vi "ViperHawk_Decode MC Data.vi"(10 "Array":u8[](array[numeric]), 11 "Diagnostic Data In":T1) -> (3 "Diagnostic Data Out":T1)   [LabVIEW 2016]
uses:
  Type Definitions/ViperHawk/ViperHawk Diagnostic Data.ctl
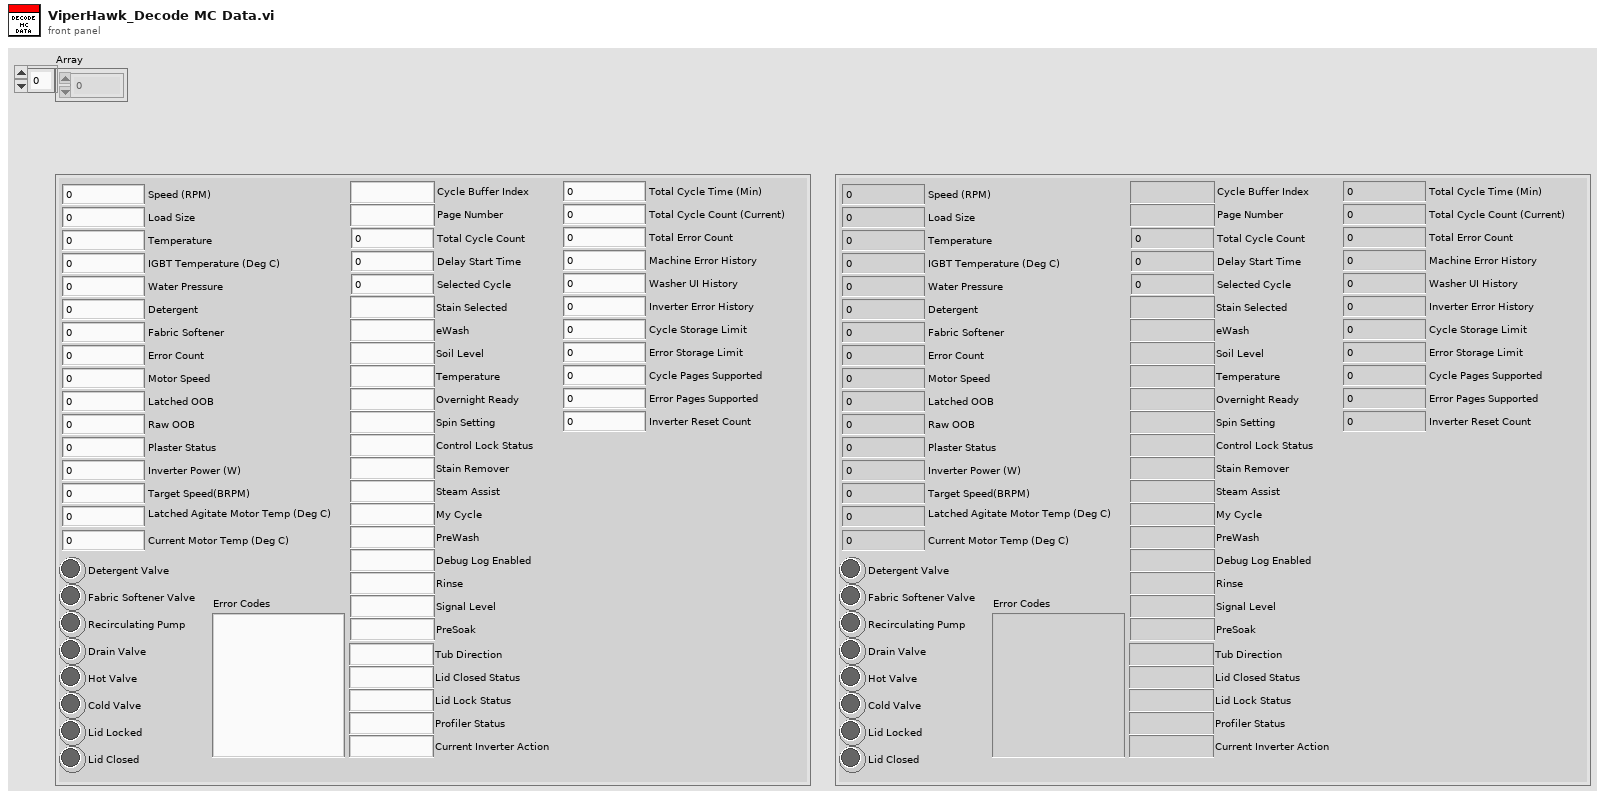
[diagram p1: front panel]
types:
  T1 = typedef "ViperHawk Diagnostic Data.ctl" = cluster{"Speed (RPM)":u32, "Load Size":u32, "Temperature":u32, "Water Pressure":dbl, "Detergent":u32, "Fabric Softener":u32, "Tub Direction":string, "Detergent Valve":bool, "Fabric Softener Valve":bool, "Recirculating Pump":bool, "Drain Valve":bool, "Hot Valve":bool, "Cold Valve":bool, "Lid Closed Status":string, "Lid Lock Status":string, "Error Count":u32, "IGBT Temperature (Deg C)":u32, "Motor Speed":u32, "Latched OOB":u32, "Raw OOB":u32, "Plaster Status":u32, "Inverter Power (W)":u32, "Target Speed(BRPM)":u32, "Latched Agitate Motor Temp (Deg C)":u32, "Current Motor Temp (Deg C)":u32, "Profiler Status":string, "Current Inverter Action":string, "Error Codes":string, "Lid Locked":bool, "Lid Closed":bool, "9E Diagnostic Data":cluster{"Total Cycle Time (Min)":u32, "Total Cycle Count (Current)":u16, "Total Error Count":u16, "Machine Error History":u32, "Washer UI History":u32, "Inverter Error History":u32, "Cycle Storage Limit":u8, "Error Storage Limit":u8, "Cycle Pages Supported":u8, "Error Pages Supported":u8, "Inverter Reset Count":u16}, "9F Diagnostic Data":cluster{"Cycle Buffer Index":string, "Page Number":string, "Total Cycle Count":u32, "Delay Start Time":u32, "Stain Selected":string, "Selected Cycle":u32, "eWash":string, "Soil Level":string, "Temperature":string, "Overnight Ready":string, "Spin Setting":string, "Control Lock Status":string, "Stain Remover":string, "Steam Assist":string, "My Cycle":string, "PreWash":string, "Debug Log Enabled":string, "Rinse":string, "Signal Level":string, "PreSoak":string}}
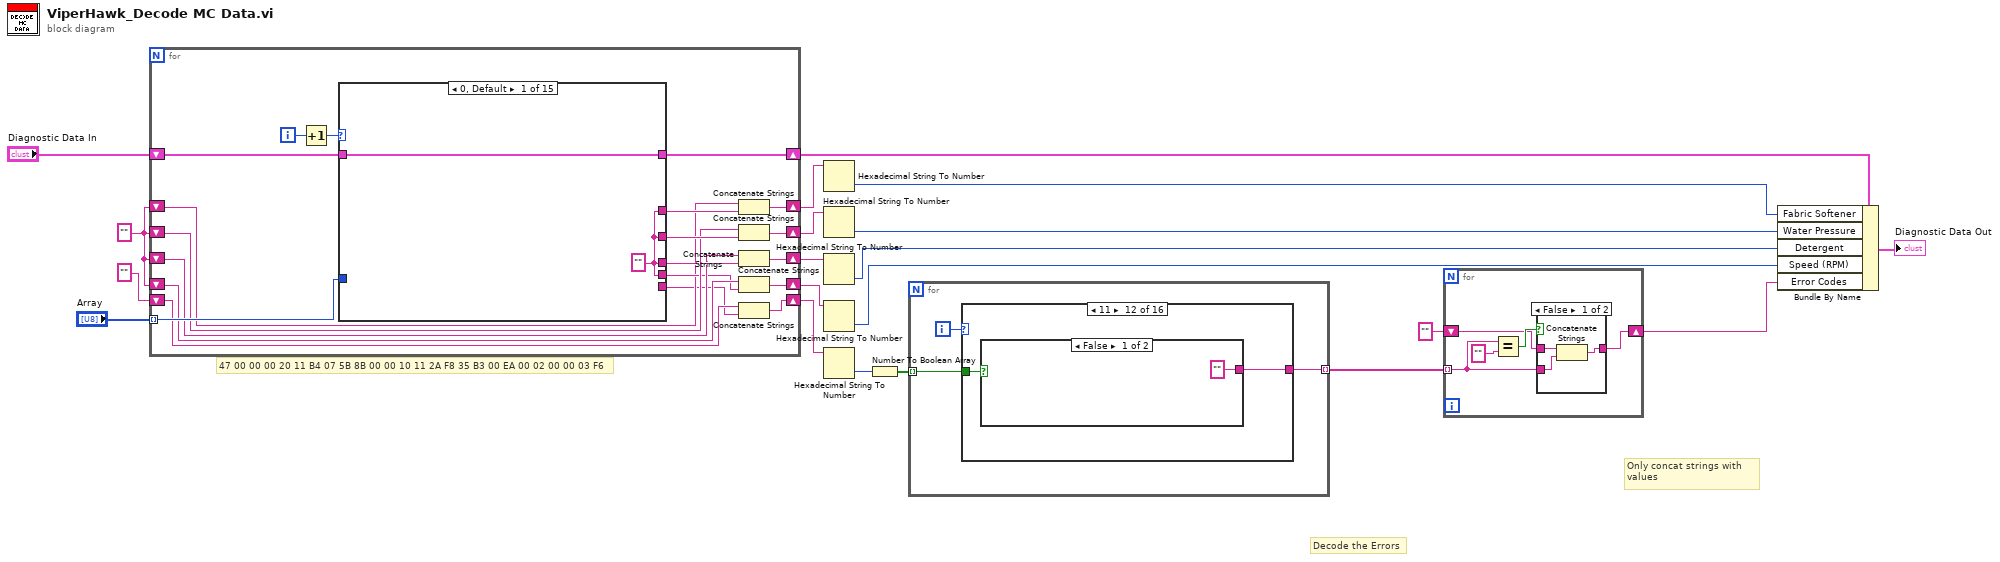
[diagram p0: block diagram]
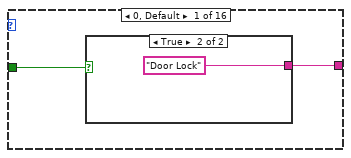
[diagram p3: hidden frame]
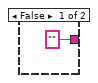
[diagram p4: hidden frame]
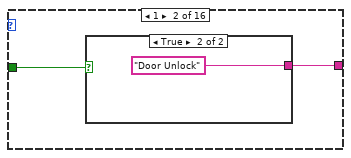
[diagram p5: hidden frame]
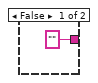
[diagram p6: hidden frame]
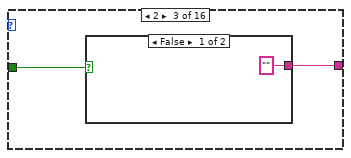
[diagram p7: hidden frame]
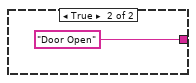
[diagram p8: hidden frame]
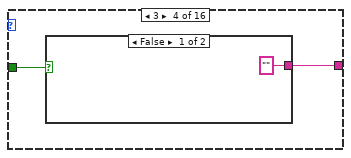
[diagram p9: hidden frame]
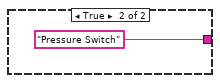
[diagram p10: hidden frame]
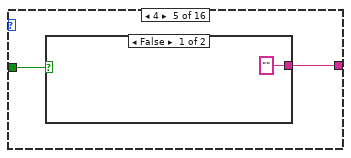
[diagram p11: hidden frame]
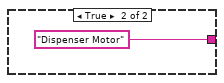
[diagram p12: hidden frame]
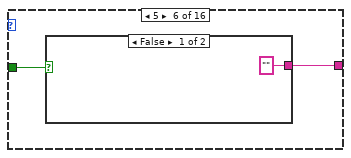
[diagram p13: hidden frame]
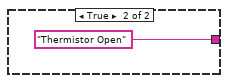
[diagram p14: hidden frame]
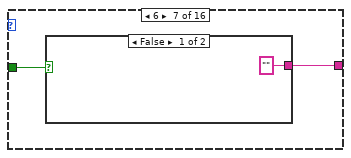
[diagram p15: hidden frame]
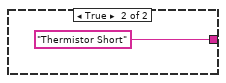
[diagram p16: hidden frame]
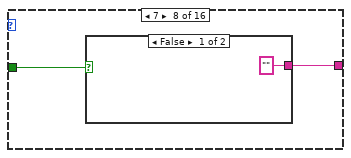
[diagram p17: hidden frame]
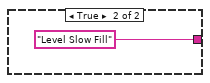
[diagram p18: hidden frame]
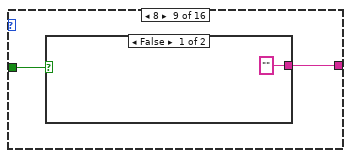
[diagram p19: hidden frame]
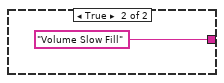
[diagram p20: hidden frame]
diagram:
  w16 = ""
  # "Only concat strings with \nvalues"
  # "Decode the Errors"
  # "47 00 00 00 20 11 B4 07 5B 8B 00 00 10 11 2A F8 35 B3 00 EA 00 02 00 00 03 F6"
  n1 = for {
    tunnel: "Array" -> [w40] mode=indexing
    shift-right: [w35] -> w19
    shift-left: w16 -> [w36]
    shift-right: [w34] -> w18
    shift-left: w16 -> [w32]
    shift-right: [w30] -> w20
    shift-left: w16 -> [w24]
    shift-right: [w29] -> w17
    shift-left: w16 -> [w28]
    shift-right: [w25] -> w15
    shift-left: "Diagnostic Data In" -> [w26]
    shift-right: [w21] -> w8
    shift-left: "" -> [w23]
    i -> [w38]
    n2 = Increment(x=w38) -> (x+1=w39:i32)
    n3 = case shown="0, Default" w39 {
      tunnel: w40 -> [_ w43 w51 w59 w63 w67 w73 w77 w80 w85 w89 w92 w96 w101 w105]
      tunnel: [w42 _ _ _ w62 w66 _ _ _ _ _ _ _ _ _] -> w37
      tunnel: [w42 _ _ _ _ _ _ w76 w79 _ _ _ _ _ _] -> w33
      tunnel: [w42 _ _ _ _ _ _ _ _ w84 w88 _ _ _ _] -> w31
      tunnel: [w42 _ _ _ _ _ _ _ _ _ _ _ _ w100 w104] -> w27
      tunnel: w26 -> [w41 w45 w49 w57 w61 w65 w71 w75 w81 w83 w87 w93 w97 w99 w103]
      tunnel: [w41 w44 w48 w56 w61 w65 w68 w75 w81 w83 w87 w93 w97 w99 w103] -> w25
      tunnel: [_ _ _ _ _ _ _ _ _ _ _ w91 w95 _ _] -> w22
      frame 0, Default {
        w42 = ""
      }
      frame 1 {
        n4 = Bundle By Name(cluster=w45, "Temperature"=w43) -> (w44:T1)
      }
      frame 4 {
        n5 = Number To Boolean Array(number=w51) -> (Boolean array=w50:bool[])
        n6 = Index Array(array=w50) -> (element #1=w47:bool, element #2=w46:bool)  [unwired: 2 in]
        n7 = Bundle By Name(cluster=w49, "Hot Valve"=w47, "Cold Valve"=w46) -> (w48:T1)
      }
      frame 5 {
        n8 = Number To Boolean Array(number=w59) -> (Boolean array=w58:bool[])
        n9 = Index Array(array=w58) -> (element #3=w55:bool, element #4=w54:bool, element #5=w53:bool, element #6=w52:bool)  [unwired: 6 in, 2 out]
        n10 = Bundle By Name(cluster=w57, "Detergent Valve"=w55, "Fabric Softener Valve"=w54, "Recirculating Pump"=w53, "Drain Valve"=w52) -> (w56:T1)
      }
      frame 6 {
        # "water pressure"
        n11 = Number To Hexadecimal String(1:i16 2 ("width (-)"), 2:w63) -> (0:w62:string)
      }
      frame 7 {
        # "water pressure"
        n12 = Number To Hexadecimal String(1:i16 2 ("width (-)"), 2:w67) -> (0:w66:string)
      }
      frame 10 {
        n13 = Number To Boolean Array(number=w73) -> (Boolean array=w72:bool[])
        n14 = Index Array(array=w72) -> (element #1=w70:bool, element #2=w69:bool)  [unwired: 2 in]
        n15 = Bundle By Name(cluster=w71, "Lid Closed"=w70, "Lid Locked"=w69) -> (w68:T1)
      }
      frame 15 {
        # "detergent"
        n16 = Number To Hexadecimal String(1:i16 2 ("width (-)"), 2:w77) -> (0:w76:string)
      }
      frame 16 {
        # "detergent"
        n17 = Number To Hexadecimal String(1:i16 2 ("width (-)"), 2:w80) -> (0:w79:string)
      }
      frame 17 {
        # "fs"
        n18 = Number To Hexadecimal String(1:i16 2 ("width (-)"), 2:w85) -> (0:w84:string)
      }
      frame 18 {
        # "fs"
        n19 = Number To Hexadecimal String(1:i16 2 ("width (-)"), 2:w89) -> (0:w88:string)
      }
      frame 21 {
        # "Error Code"
        n20 = Number To Hexadecimal String(1:i16 2 ("width (-)"), 2:w92) -> (0:w91:string)
      }
      frame 22 {
        # "Error Code"
        n21 = Number To Hexadecimal String(1:i16 2 ("width (-)"), 2:w96) -> (0:w95:string)
      }
      frame 25 {
        # "hall sensor"
        n22 = Number To Hexadecimal String(1:i16 2 ("width (-)"), 2:w101) -> (0:w100:string)
      }
      frame 26 {
        # "hall sensor"
        n23 = Number To Hexadecimal String(1:i16 2 ("width (-)"), 2:w105) -> (0:w104:string)
      }
    }
    n24 = Concatenate Strings(w24, w31) -> (w30:string)
    n25 = Concatenate Strings(w36, w37) -> (w35:string)
    n26 = Concatenate Strings(w32, w33) -> (w34:string)
    n27 = Concatenate Strings(w28, w27) -> (w29:string)
    n28 = Concatenate Strings(w23, w22) -> (w21:string)
  }
  n29 = Hexadecimal String To Number(string=w20) -> (number=w12:u32)  [unwired: 2 in, 1 out]
  n30 = Hexadecimal String To Number(string=w19) -> (number=w13:u32)  [unwired: 2 in, 1 out]
  n31 = Hexadecimal String To Number(string=w18) -> (number=w14:u32)  [unwired: 2 in, 1 out]
  n32 = Hexadecimal String To Number(string=w17) -> (number=w11:u32)  [unwired: 2 in, 1 out]
  n33 = Hexadecimal String To Number(string=w8) -> (number=w7:u32)  [unwired: 2 in, 1 out]
  n34 = Number To Boolean Array(number=w7) -> (Boolean array=w10:bool[])
  n35 = for {
    tunnel: w10 -> [w107] mode=indexing
    tunnel: [w106] -> w6 mode=indexing
    i -> [w108]
    n36 = case shown="11" w108 {
      tunnel: w107 -> [w110 w114 w118 w122 w126 w130 w134 w138 w141 w145 w149 w153 w157 w161 _ _]
      tunnel: [w109 w113 w117 w121 w125 w129 w133 w137 w142 w146 w150 w154 w158 w162 "" ""] -> w106
      frame 0, Default {
        n37 = case shown="True" w110 {
          tunnel: ["" "Door Lock"] -> w109
          frame False {
          }
          frame True {
          }
        }
      }
      frame 1 {
        n38 = case shown="True" w114 {
          tunnel: ["" "Door Unlock"] -> w113
          frame False {
          }
          frame True {
          }
        }
      }
      frame 2 {
        n39 = case shown="False" w118 {
          tunnel: ["" "Door Open"] -> w117
          frame False {
          }
          frame True {
          }
        }
      }
      frame 3 {
        n40 = case shown="False" w122 {
          tunnel: ["" "Pressure Switch"] -> w121
          frame False {
          }
          frame True {
          }
        }
      }
      frame 4 {
        n41 = case shown="False" w126 {
          tunnel: ["" "Dispenser Motor"] -> w125
          frame False {
          }
          frame True {
          }
        }
      }
      frame 5 {
        n42 = case shown="False" w130 {
          tunnel: ["" "Thermistor Open"] -> w129
          frame False {
          }
          frame True {
          }
        }
      }
      frame 6 {
        n43 = case shown="False" w134 {
          tunnel: ["" "Thermistor Short"] -> w133
          frame False {
          }
          frame True {
          }
        }
      }
      frame 7 {
        n44 = case shown="False" w138 {
          tunnel: ["" "Level Slow Fill"] -> w137
          frame False {
          }
          frame True {
          }
        }
      }
      frame 8 {
        n45 = case shown="False" w141 {
          tunnel: ["" "Volume Slow Fill"] -> w142
          frame False {
          }
          frame True {
          }
        }
      }
      frame 9 {
        n46 = case shown="False" w145 {
          tunnel: ["" "Drain System"] -> w146
          frame False {
          }
          frame True {
          }
        }
      }
      frame 10 {
        n47 = case shown="False" w149 {
          tunnel: ["" "EEPROM"] -> w150
          frame False {
          }
          frame True {
          }
        }
      }
      frame 11 {
        n48 = case shown="False" w153 {
          tunnel: ["" "Target Volume Overflow"] -> w154
          frame False {
          }
          frame True {
          }
        }
      }
      frame 12 {
        n49 = case shown="False" w157 {
          tunnel: ["" "Overflow"] -> w158
          frame False {
          }
          frame True {
          }
        }
      }
      frame 13 {
        n50 = case shown="True" w161 {
          tunnel: ["" "Inverter Redundancy"] -> w162
          frame False {
          }
          frame True {
          }
        }
      }
      frame 14 {
      }
      frame 15 {
      }
    }
  }
  n51 = for {
    tunnel: w6 -> [w168] mode=indexing
    shift-right: [w167] -> w4
    shift-left: "" -> [w169]
    n52 = Equal?(x=w168, y="") -> (x = y?=w170:bool)
    n53 = case shown="False" w170 {
      tunnel: w169 -> [w174 w175]
      tunnel: w168 -> [w173 _]
      tunnel: [w172 w175] -> w167
      frame False {
        n54 = Concatenate Strings(w174, w173) -> (w172:string)
      }
      frame True {
      }
    }
  }
  n55 = Bundle By Name(cluster=w15, "Fabric Softener"=w12, "Water Pressure"=w13, "Detergent"=w14, "Speed (RPM)"=w11, "Error Codes"=w4) -> (→"Diagnostic Data Out":T1)
